vi "MSO9104B_RunAndGetDigitalWaveformData.vi"(7 "Maximum Time (10000ms)":u32=10000, 8 "error in (no error)":errorcluster, 9 "Segment Index (0)":i32 format="%.0g", 10 "Channel (41: POD 1)":i32(ring)=41 items=["POD 1"=41, "POD 2"=42], 11 "VISA resource name":refnum<visa-resource-name>) -> (0 "error out":errorcluster, 1 "min value":i8, 2 "max value":i8, 3 "VISA resource name out":refnum<visa-resource-name>)   [LabVIEW 2016]
uses:
  <userlib>/_TI-LA/Instr Drivers/Oscilloscope/MSO9104A/Driver/Base/Agilent 90000 Series/Agilent 90000 Series.lvlib
panel:
  out "DataArray":i8[](array[numeric])
  out "Digital Waveform Graph":digitalwaveform(graph)
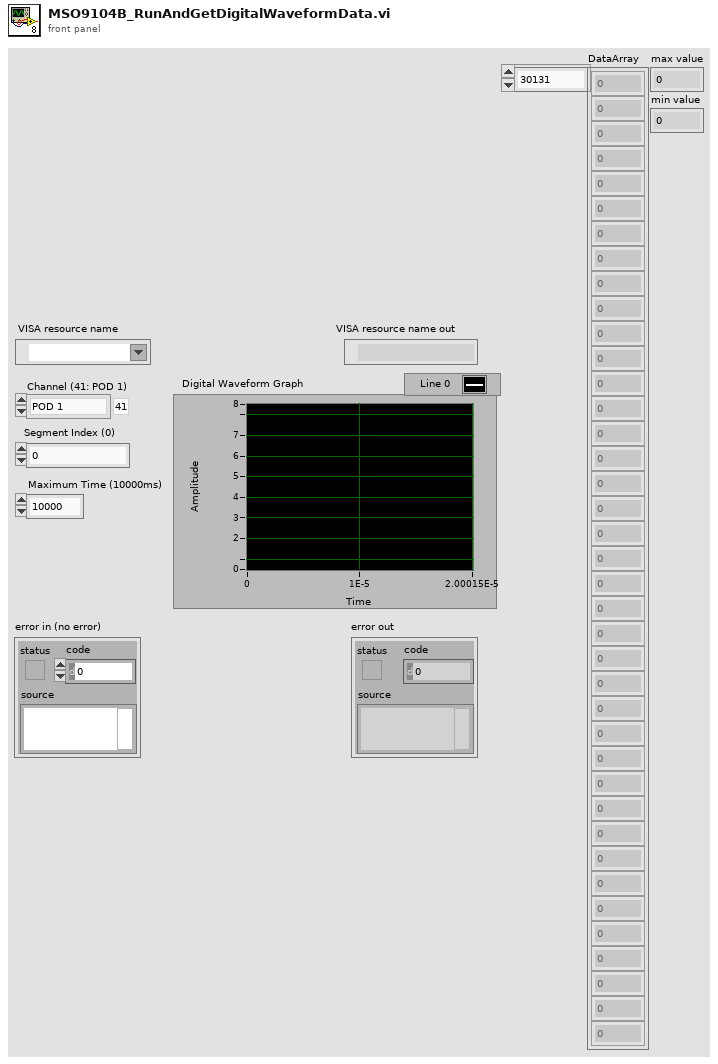
[diagram p1: front panel]
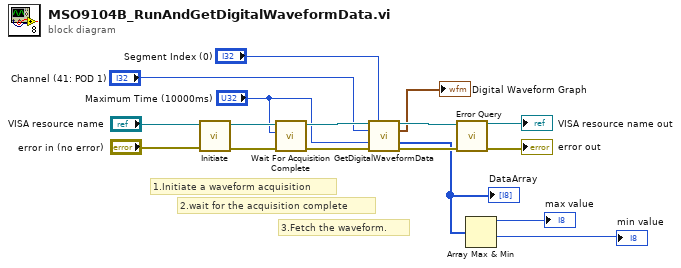
[diagram p0: block diagram]
diagram:
  # "3.Fetch the waveform."
  # "2.wait for the acquisition complete"
  # "1.Initiate a waveform acquisition"
  n1 = call <userlib>:"Initiate.vi"("error in (no error)"="error in (no error)", "VISA resource name"="VISA resource name") -> ("error out"=w12:errorcluster, "VISA resource name out"=w13:refnum<visa-resource-name>)  [unwired: 8 out]
  n2 = call <userlib>:"Wait For Acquisition Complete.vi"("error in (no error)"=w12, "Maximum Time (10000ms)"="Maximum Time (10000ms)", "VISA resource name"=w13) -> ("error out"=w8:errorcluster, "VISA resource name out"=w9:refnum<visa-resource-name>)  [unwired: 7 out]
  n3 = call "GetDigitalWaveformData.vi"("VISA resource name"=w9, "Segment Index (0)"="Segment Index (0)", "Channel (41: POD 1)"="Channel (41: POD 1)", "Maximum Time (10000ms)"="Maximum Time (10000ms)", "error in (no error)"=w8) -> ("VISA resource name out"=w10:refnum<visa-resource-name>, "Digital Waveform Graph"=→"Digital Waveform Graph":digitalwaveform, "Array"=w3:i8[], "error out"=w11:errorcluster)  [unwired: 7 in]
  "DataArray" <- w3
  n4 = call <userlib>:"Error Query.vi"("error in (no error)"=w11, "VISA resource name"=w10) -> ("error out"=→"error out":errorcluster, "VISA resource name out"=→"VISA resource name out":refnum<visa-resource-name>)  [unwired: 8 out]
  n5 = Array Max & Min(array=w3) -> (max value=→"max value":i8, min value=→"min value":i8)  [unwired: 2 out]
